vi "QBPN-Create.vi"(0 "Filter":T1 {"IIR Filter Cluster"."Forward Coefficients" format="%.4f"; "IIR Filter Cluster"."Reverse Coefficients" format="%.4f"}, 7 "Npts":i32=128, 11 "Omega (t)":dbl[](array[numeric])) -> (4 "Filter (out)":T1 {"IIR Filter Cluster"."Forward Coefficients" format="%.4f"; "IIR Filter Cluster"."Reverse Coefficients" format="%.4f"}, 8 "BP noise":dbl[](array[numeric]))   [LabVIEW 2015]
doc: "Create a token of bandpass noise using the quadrature filter method."
uses:
  Controls/Filter XCtl/Filter Data.ctl
  <vilib>/Analysis/3filter.llb/IIR Cascade Filter with I.C. (DBL).vi
  <vilib>/Analysis/NI_AALBase.lvlib
  Controls/Filter XCtl/Filter XCtl.xctl
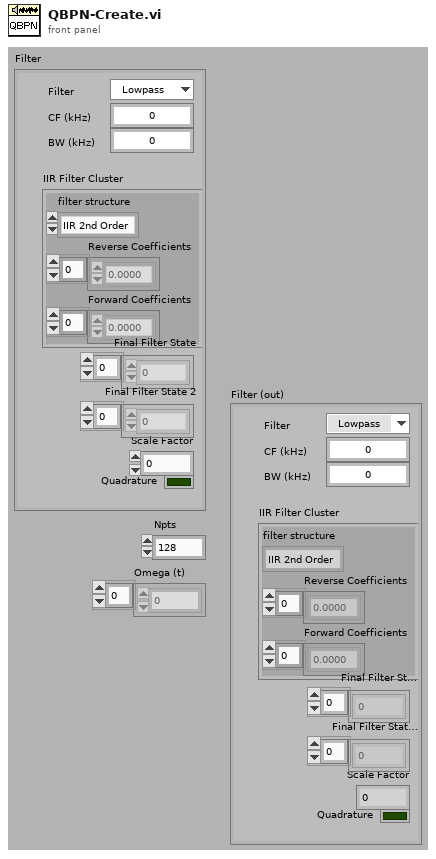
[diagram p1: front panel]
types:
  T1 = typedef "Filter XCtl.xctl/Filter Data.ctl" = cluster{"CF (kHz)":dbl, "BW (kHz)":dbl, "IIR Filter Cluster":cluster{"filter structure":enum32{"IIR 2nd Order", "IIR 4th Order"}, "Reverse Coefficients":dbl[], "Forward Coefficients":dbl[]}, "Final Filter State":dbl[], "Scale Factor":dbl, "Final Filter State 2":dbl[], "Quadrature":bool, "Type":enum16{"Lowpass", "Highpass", "Bandpass", "Bandstop", "OFF"}}
  T2 = cluster{"filter structure":enum32{"IIR 2nd Order", "IIR 4th Order"}, "Reverse Coefficients":dbl[], "Forward Coefficients":dbl[]}
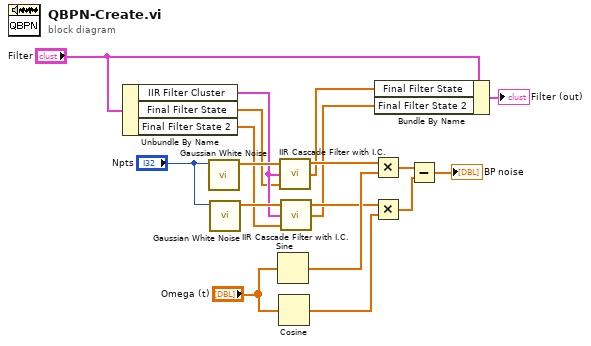
[diagram p0: block diagram]
diagram:
  n1 = Unbundle By Name("Filter") -> ("IIR Filter Cluster"=w7:T2, "Final Filter State"=w6:dbl[], "Final Filter State 2"=w5:dbl[])
  n2 = call <vilib>:"Gaussian White Noise.vi"("samples"="Npts") -> ("Gaussian noise pattern"=w17:dbl[])  [unwired: 9 in, 1 out]
  n3 = call <vilib>:"Gaussian White Noise.vi"("samples"="Npts") -> ("Gaussian noise pattern"=w18:dbl[])  [unwired: 9 in, 1 out]
  n4 = Sine(x="Omega (t)") -> (sin(x)=w16:dbl[])
  n5 = Cosine(x="Omega (t)") -> (cos(x)=w14:dbl[])
  n6 = call-poly <vilib>:"IIR Cascade Filter with I.C..vi"("Initial Filter State"=w6, "IIR Filter Cluster"=w7, "X"=w17) -> ("Final Filter State"=w3:dbl[], "Filtered X"=w11:dbl[])  [unwired: 1 out]
  n7 = call-poly <vilib>:"IIR Cascade Filter with I.C..vi"("Initial Filter State"=w5, "IIR Filter Cluster"=w7, "X"=w18) -> ("Final Filter State"=w2:dbl[], "Filtered X"=w15:dbl[])  [unwired: 1 out]
  n8 = Multiply(x=w11, y=w16) -> (x*y=w13:dbl[])
  n9 = Multiply(x=w15, y=w14) -> (x*y=w12:dbl[])
  n10 = Bundle By Name(cluster="Filter", "Final Filter State"=w3, "Final Filter State 2"=w2) -> (→"Filter (out)":T1)
  n11 = Subtract(x=w13, y=w12) -> (x-y=→"BP noise":dbl[])
